vi "SETPINSTATUS.vi"(0 "simulado in":refnum<class "simulado.lvclass">, 5 "PORT":dbl, 7 "PIN":dbl, 9 "valor":bool, 11 "error in (no error)":errorcluster) -> (4 "simulado out":refnum<class "simulado.lvclass">, 15 "error out":errorcluster)   [LabVIEW 2019, in "simulado.lvclass"]
uses:
  simulado.lvclass
  simulado.lvclass/simulado.ctl
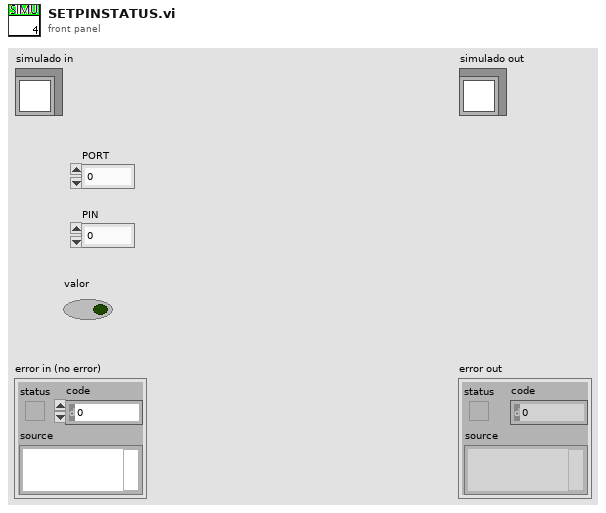
[diagram p1: front panel]
types:
  T1 = enum16{"get parameter", "Set parameters", "reset parameter", ""}
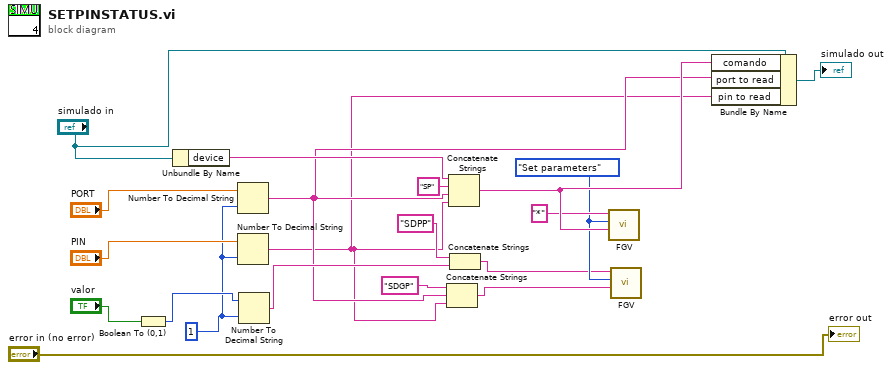
[diagram p0: block diagram]
diagram:
  w9 = T1."Set parameters" ("functions")
  w16 = i16 1 ("width (-)")
  n1 = Boolean To (0,1)(Boolean="valor") -> (0, 1=w17:i16)
  n2 = Unbundle By Name("simulado in") -> ("device"=w12:string)
  n3 = Number To Decimal String(number="PORT", width (-)=w16) -> (decimal integer string=w2:string)
  n4 = Number To Decimal String(number="PIN", width (-)=w16) -> (decimal integer string=w1:string)
  n5 = Number To Decimal String(number=w17, width (-)=w16) -> (decimal integer string=w6:string)
  n6 = Concatenate Strings("SDGP" ("string"), w2, w1) -> (w4:string)
  n7 = Concatenate Strings(w12, "SP" ("string"), w2, w1) -> (w11:string)
  n8 = Concatenate Strings("SDPP" ("string"), w6) -> (w5:string)
  n9 = call "FGV.vi"("command"=w11, "functions"=w9, "response to save"="*") -> ()  [unwired: 7 in, 2 out]
  n10 = call "FGV.vi"("command"=w4, "functions"=w9, "response to save"=w5) -> ()  [unwired: 7 in, 2 out]
  n11 = Bundle By Name(cluster="simulado in", "comando"=w11, "port to read"=w2, "pin to read"=w1) -> (→"simulado out":refnum<class "simulado.lvclass">)
  "error out" <- "error in (no error)"
